vi "UDP 읽기.vi"() -> ()   [LabVIEW 2014]
panel:
  in  "정지":bool
  out "웨이브폼 그래프":dbl[](graph)
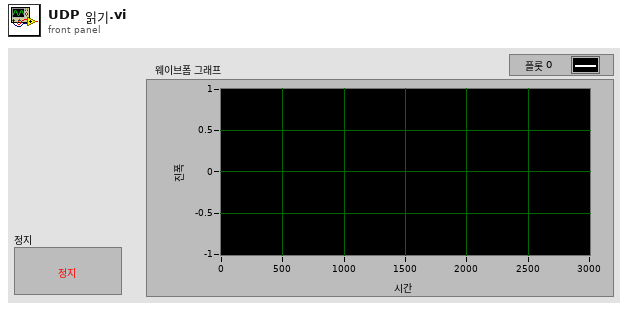
[diagram p1: front panel]
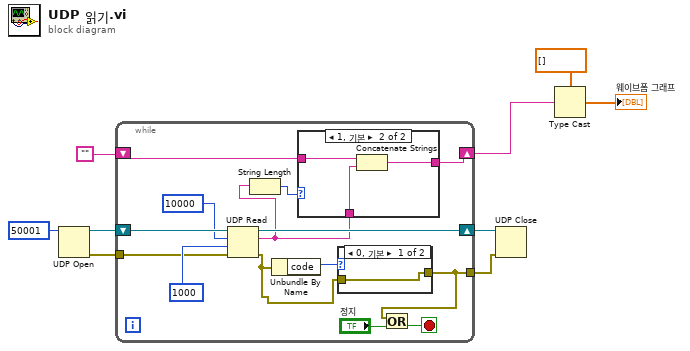
[diagram p0: block diagram]
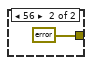
[diagram p2: hidden frame]
diagram:
  n1 = UDP Open(11:u16 50001 ("포트")) -> (port=w9:refnum<k16>, 0:w2:errorcluster)  [unwired: 4 in, 1 out]
  n2 = while {
    shift-right: [w22] -> w8
    shift-left: w9 -> [w23]
    shift-right: [w18] -> w3
    shift-left: "" -> [w19]
    tunnel: w2 -> [w14]
    tunnel: [w10] -> w1
    stop <- w11 stop-if-true
    n3 = UDP Read(connection ID=w23, max size (548)=10000 ("최대 크기(548)"), timeout ms (25000)=1000 ("타임아웃 ms (25000)"), 8:w14) -> (data out=w17:string, error out=w12:errorcluster, 3:w22:refnum<k16>)  [unwired: 2 out]
    n4 = String Length(string=w17) -> (length=w16:i32)
    n5 = Unbundle By Name(w12) -> ("code"=w13:i32)
    n6 = case shown="1, 기본" w16 {
      tunnel: w19 -> [w26 w29]
      tunnel: [w26 w28] -> w18
      tunnel: w17 -> [_ w27]
      frame 0 {
      }
      frame 1, Default {
        n7 = Concatenate Strings(w29, w27) -> (w28:string)
      }
    }
    n8 = case shown="0, 기본" w13 {
      tunnel: [w24 errorcluster {"status"=FALSE, "code"=0, "source"=""} ("에러 상수")] -> w10
      tunnel: w12 -> [w24 _]
      frame 0, Default {
      }
      frame 56 {
      }
    }
    n9 = Or(x=w10, y="정지") -> (x .or. y?=w11:bool)
  }
  n10 = UDP Close(connection ID=w8, 8:w1) -> ()  [unwired: 2 out]
  n11 = Type Cast(type=dbl[] [], x=w3) -> (*(type *) &x=→"웨이브폼 그래프":dbl[])
